vi "East Window Control.vi"() -> (0 "Error string":string)   [LabVIEW 2022 SP3]
uses:
  Anemometry/Anemometry Sub Vis/Globals/Dynamic_call_global.ph.vi
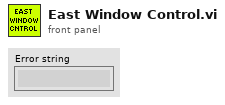
[diagram p1: front panel]
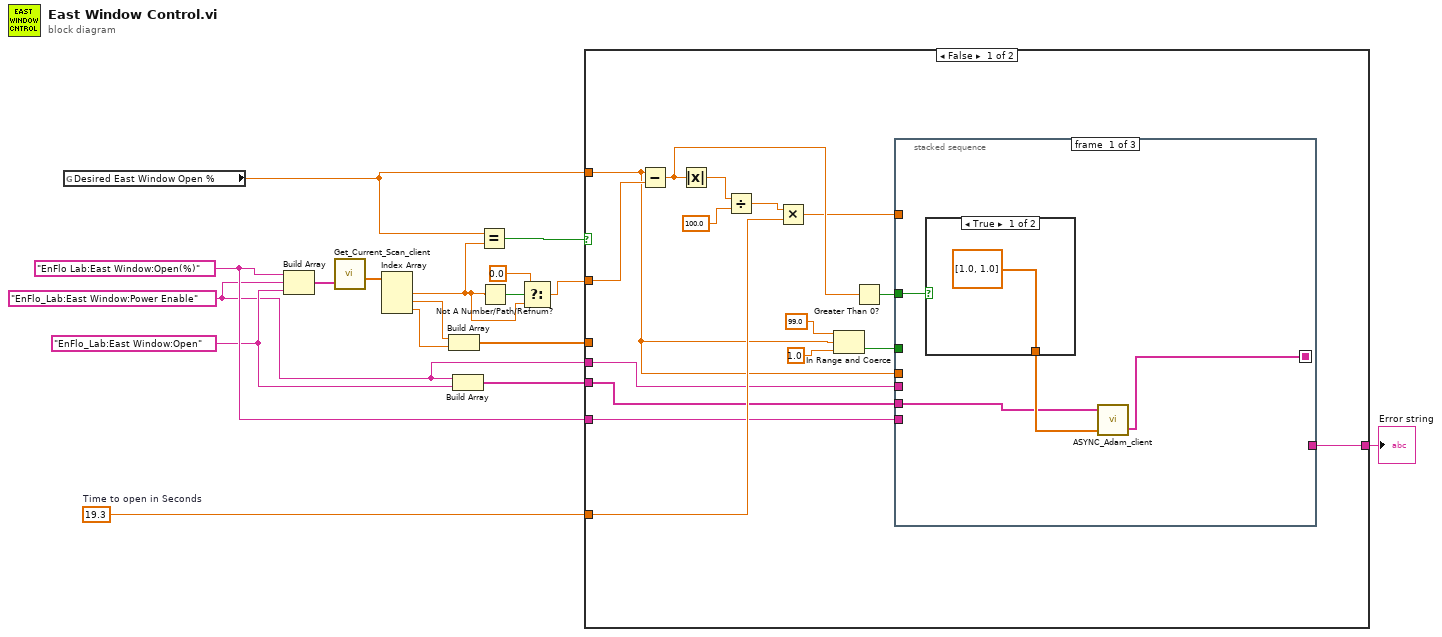
[diagram p0: block diagram]
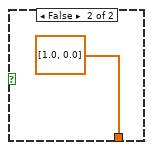
[diagram p2: hidden frame]
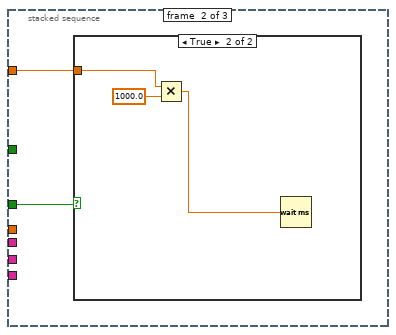
[diagram p3: hidden frame]
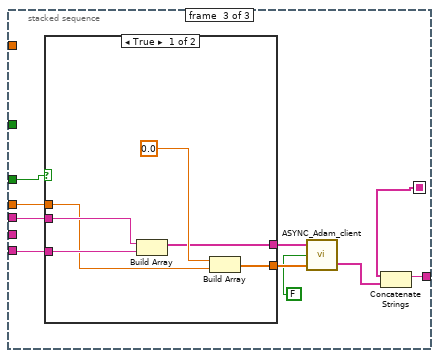
[diagram p5: hidden frame]
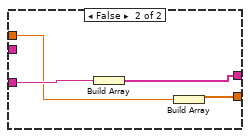
[diagram p6: hidden frame]
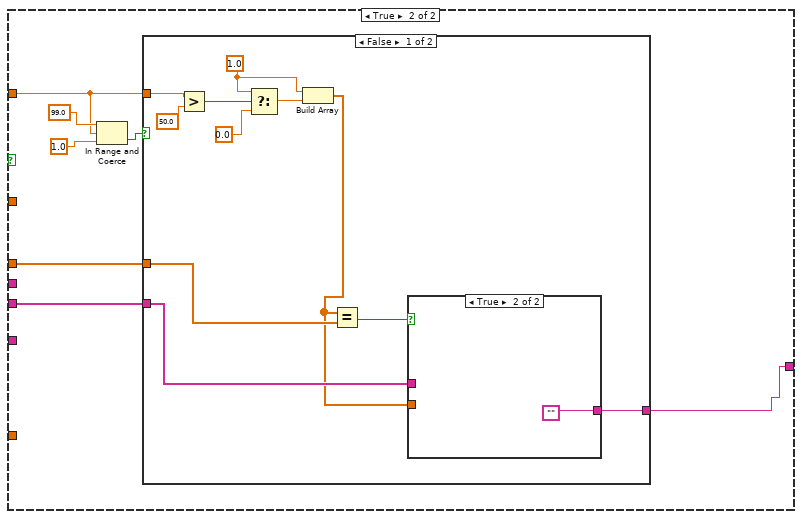
[diagram p7: hidden frame]
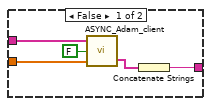
[diagram p8: hidden frame]
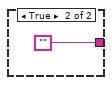
[diagram p9: hidden frame]
diagram:
  w3 = "EnFlo_Lab:East Window:Open"
  w1 = "EnFlo_Lab:East Window:Power Enable"
  w14 = 19.3  # Time to open in Seconds
  w13 = "EnFlo Lab:East Window:Open(%)"
  n1 = global read "Dynamic_call_global.ph.vi" "Desired East Window Open %"() -> (w7:dbl)
  n2 = Build Array(w13, w1, w3) -> (w17:string[])
  n3 = call "Get_Current_Scan_client.vi"("multipleChannels"=w17) -> ("Numerical Values"=w16:dbl[])  [unwired: 1 in, 3 out]
  n4 = Index Array(array=w16) -> (element #1=w8:dbl, element #2=w6:dbl, element #3=w5:dbl)  [unwired: 3 in]
  n5 = Build Array(w6, w5) -> (w4:dbl[])
  n6 = Build Array(w1, w3) -> (w2:string[])
  n7 = Equal?(x=w7, y=w8) -> (x = y?=w15:bool)
  n8 = Not A Number/Path/Refnum?(number/path/refnum=w8) -> (NaN/Path/Refnum?=w11:bool)
  n9 = Select(t=0.0, s=w11, f=w8) -> (s? t:f=w10:dbl)
  n10 = case shown="False" w15 {
    tunnel: w7 -> [w24 w68]
    tunnel: w10 -> [w33 _]
    tunnel: w14 -> [w30 _]
    tunnel: w13 -> [w25 _]
    tunnel: [w23 w65] -> w12
    tunnel: w4 -> [_ w67]
    tunnel: w2 -> [w19 w66]
    tunnel: w1 -> [w18 _]
    frame False {
      n11 = Subtract(x=w24, y=w33) -> (x-y=w28:dbl)
      n12 = Absolute Value(x=w28) -> (abs(x)=w29:dbl)
      n13 = Divide(x=w29, y=100.0) -> (x/y=w31:dbl)
      n14 = Multiply(x=w31, y=w30) -> (x*y=w26:dbl)
      n15 = In Range and Coerce(upper limit=99.0, x=w24, lower limit=1.0) -> (In Range?=w20:bool)  [unwired: 1 out]
      n16 = Greater Than 0?(x=w28) -> (x > 0?=w27:bool)
      n17 = stacked-sequence {
        seq-local: [w35 _ _] -> [_ _ w49]
        tunnel: w27 -> [w37 _ _]
        tunnel: w26 -> [_ w41 _]
        tunnel: w18 -> [_ _ w54]
        tunnel: w25 -> [_ _ w53]
        tunnel: w24 -> [_ _ w52]
        tunnel: [_ _ w46] -> w23
        tunnel: w20 -> [_ w40 w51]
        tunnel: w19 -> [w34 _ _]
        frame #0 {
          n18 = case shown="True" w37 {
            tunnel: [dbl[] [1.0, 1.0] ("Values") dbl[] [1.0, 0.0] ("Values")] -> w36
            frame True {
            }
            frame False {
            }
          }
          n19 = call "ASYNC_Adam_client.vi"("Values"=w36, "Channel Names"=w34) -> ("Scan Comments"=w35:string[])  [unwired: 1 in, 1 out]
        }
        frame #1 {
          n20 = case shown="True" w40 {
            tunnel: w41 -> [_ w44]
            frame False {
            }
            frame True {
              n21 = Multiply(x=w44, y=1000.0) -> (x*y=w42:dbl)
              n22 = Wait (ms)(milliseconds to wait=w42) -> ()  [unwired: 1 out]
            }
          }
        }
        frame #2 {
          n23 = case shown="True" w51 {
            tunnel: w54 -> [w60 _]
            tunnel: w53 -> [w58 w64]
            tunnel: w52 -> [w57 w63]
            tunnel: [w56 w62] -> w48
            tunnel: [w55 w61] -> w47
            frame True {
              n24 = Build Array(w60, w58) -> (w56:string[])
              n25 = Build Array(0.0, w57) -> (w55:dbl[])
            }
            frame False {
              n26 = Build Array(w64) -> (w62:string[])
              n27 = Build Array(w63) -> (w61:dbl[])
            }
          }
          n28 = call "ASYNC_Adam_client.vi"("Values"=w47, "Check Value is in the scan table?"=FALSE, "Channel Names"=w48) -> ("Scan Comments"=w50:string[])  [unwired: 1 out]
          n29 = Concatenate Strings(w49, w50) -> (w46:string)
        }
      }
    }
    frame True {
      n30 = In Range and Coerce(upper limit=99.0, x=w68, lower limit=1.0) -> (In Range?=w69:bool)  [unwired: 1 out]
      n31 = case shown="False" w69 {
        tunnel: w68 -> [w82 _]
        tunnel: w67 -> [w80 _]
        tunnel: w66 -> [w78 _]
        tunnel: [w72 ""] -> w65
        frame False {
          w74 = 1.0 ("t")
          n32 = Greater?(x=w82, y=50.0) -> (0:w77:bool)
          n33 = Select(t=w74, s=w77, f=0.0) -> (s? t:f=w75:dbl)
          n34 = Build Array(w74, w75) -> (w73:dbl[])
          n35 = Equal?(x=w73, y=w80) -> (x = y?=w79:bool)
          n36 = case shown="True" w79 {
            tunnel: w78 -> [w87 _]
            tunnel: w73 -> [w86 _]
            tunnel: [w83 ""] -> w72
            frame False {
              n37 = call "ASYNC_Adam_client.vi"("Values"=w86, "Check Value is in the scan table?"=FALSE, "Channel Names"=w87) -> ("Scan Comments"=w84:string[])  [unwired: 1 out]
              n38 = Concatenate Strings(w84) -> (w83:string)
            }
            frame True {
            }
          }
        }
        frame True {
        }
      }
    }
  }
  "Error string" <- w12
